vi "RDS Load Config.vi"() -> (3 "RDS Config":T1={"State Update Rate (Hz)"=0.0, "Helm Rate (Hz)"=0.0, "Helm Gains"={"P (Kc)"=0.0, "I (Ti)"=0.0, "D (Td)"=0.0}, "Limiter"=100.0, "Mission Controller Settings"={"Waypoint Radius (m)"=0.0}, "Mag Dev"=0.0} {"Helm Gains"."D (Td)" format="%#_9f"; "Helm Gains"."I (Ti)" format="%#_9f"; "Helm Gains"."P (Kc)" format="%#.9f"})   [LabVIEW 2015, in "RDS Configuration Library.lvlib"]
uses:
  RDS Configuration Library.lvlib
  RDS Configuration.ctl
  RDS Child Messages/PID Gains/PID Gains Control.ctl
  RDS Mission Controller Actor/Mission Controller Settings.ctl
  RDS Child Messages/RDS Child Messages.lvlib
  RDS Mission Controller Actor/RDS Mission Controller Actor.lvlib
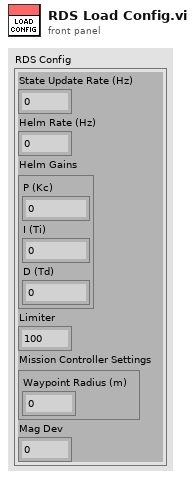
[diagram p1: front panel]
types:
  T1 = typedef "RDS Configuration Library.lvlib/RDS Configuration.ctl" = cluster{"State Update Rate (Hz)":dbl, "Helm Rate (Hz)":dbl, "Helm Gains":T2, "Limiter":dbl, "Mission Controller Settings":T3, "Mag Dev":dbl}
  T2 = typedef "RDS Child Messages.lvlib/PID Gains Control.ctl" = cluster{"P (Kc)":sgl, "I (Ti)":sgl, "D (Td)":sgl}
  T3 = typedef "RDS Mission Controller Actor.lvlib/Mission Controller Settings.ctl" = cluster{"Waypoint Radius (m)":dbl}
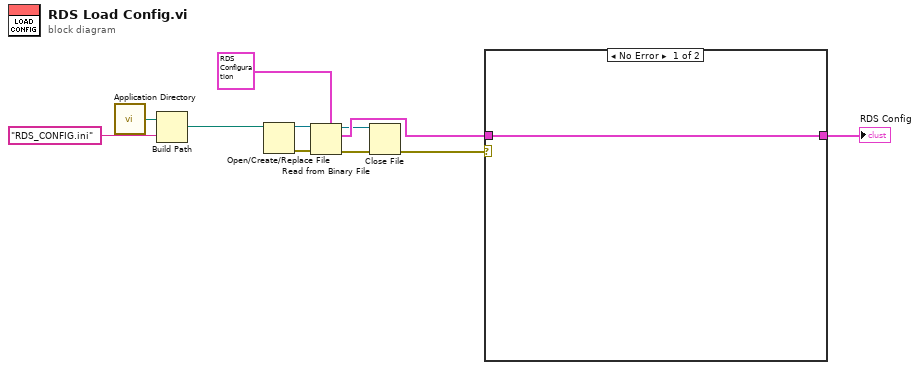
[diagram p0: block diagram]
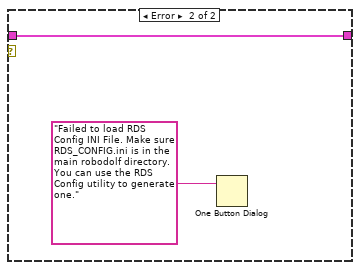
[diagram p2: hidden frame]
diagram:
  n1 = call <vilib>:"Application Directory.vi"() -> ("Application Directory"=w11:path)
  n2 = Build Path(base path=w11, name or relative path="RDS_CONFIG.ini") -> (appended path=w2:path)
  n3 = Open/Create/Replace File(file path (use dialog)=w2) -> (refnum out=w3:refnum<file>, error out=w4:errorcluster)  [unwired: 5 in, 1 out]
  n4 = Read from Binary File(5:T1 {"State Update Rate (Hz)"=0.0, "Helm Rate (Hz)"=0.0, "Helm Gains"={"P (Kc)"=0.0, "I (Ti)"=0.0, "D (Td)"=0.0}, "Limiter"=100.0, "Mission Controller Settings"={"Waypoint Radius (m)"=0.0}, "Mag Dev"=0.0} ("RDS Config"), 8:w4, 11:w3) -> (0:w5:errorcluster, 2:w8:T1, 3:w6:refnum<file>)  [unwired: 3 in, 1 out]
  n5 = Close File(refnum=w6, error in=w5) -> (error out=w1:errorcluster)  [unwired: 1 out]
  n6 = case shown="No Error" w1 {
    tunnel: [w12 w13] -> w7
    tunnel: w8 -> [w12 w13]
    frame No Error {
    }
    frame Error {
      n7 = One Button Dialog(message="Failed to load RDS Config INI File. Make sure RDS_CONFIG.ini is in the main robodolf directory. You can use the RDS Config utility to generate one.") -> ()  [unwired: 1 in, 1 out]
    }
  }
  "RDS Config" <- w7
